vi "PlotOHparams.vi"() -> ()   [LabVIEW 2014]
uses:
  Slicer_11-28/LVslicer/Slice/TypeDefs/RectHatch.ctl
  Slicer_11-28/LVslicer/Slice/TypeDefs/PowerSpeed.ctl
  Slicer_11-28/LVslicer/Slice/TypeDefs/Area PWRMap Params.ctl
  <vilib>/picture/3D Picture Control/Object/Create Object (name).vi
  <vilib>/Utility/file.llb/Read From Spreadsheet File (DBL).vi
  <vilib>/picture/3D Picture Control/NI_3D Picture Control.lvlib
panel:
  out "Array":T1[](array[typedef])
  out "Layer":dbl
  in  "stop":bool
  out "3D Picture":refnum<vi>(3d-picture)
  out "OH":T2(array[cluster])=[{-30.0, 30.0, 382.0, 300.0, 114.6, 229.2, 229.2, 382.0, 382.0}, {-15.0, 30.0, 382.0, 300.0, 95.5, 191.0, 286.5, 382.0, 382.0}, {0.0, 30.0, 327.0, 150.0, 98.1, 196.2, 196.2, 327.0, 327.0}, {15.0, 30.0, 382.0, 300.0, 114.6, 229.2, 229.2, 382.0, 382.0}, {30.0, 30.0, 382.0, 300.0, 152.8, 191.0, 229.2, 267.4, 382.0}, {-30.0, 15.0, 382.0, 300.0, 95.5, 191.0, 286.5, 382.0, 382.0}, {-15.0, 15.0, 327.0, 150.0, 81.75, 163.5, 245.25, 327.0, 327.0}, {0.0, 15.0, 382.0, 300.0, 152.8, 191.0, 229.2, 267.4, 382.0}, {15.0, 15.0, 327.0, 150.0, 130.8, 163.5, 196.2, 228.9, 327.0}, {30.0, 15.0, 382.0, 300.0, 114.6, 229.2, 229.2, 382.0, 382.0}, {-30.0, 0.0, 327.0, 150.0, 98.1, 196.2, 196.2, 327.0, 327.0}, {-15.0, 0.0, 382.0, 300.0, 95.5, 191.0, 286.5, 382.0, 382.0}, {0.0, 0.0, 327.0, 150.0, 81.75, 163.5, 245.25, 327.0, 327.0}, {15.0, 0.0, 382.0, 300.0, 152.8, 191.0, 229.2, 267.4, 382.0}, {30.0, 0.0, 327.0, 150.0, 130.8, 163.5, 196.2, 228.9, 327.0}, {-30.0, -15.0, 382.0, 300.0, 114.6, 229.2, 229.2, 382.0, 382.0}, {-15.0, -15.0, 327.0, 150.0, 98.1, 196.2, 196.2, 327.0, 327.0}, {0.0, -15.0, 382.0, 300.0, 95.5, 191.0, 286.5, 382.0, 382.0}, {15.0, -15.0, 327.0, 150.0, 81.75, 163.5, 245.25, 327.0, 327.0}, {30.0, -15.0, 382.0, 300.0, 152.8, 191.0, 229.2, 267.4, 382.0}, {-30.0, -30.0, 382.0, 300.0, 114.6, 229.2, 229.2, 382.0, 382.0}, {-15.0, -30.0, 382.0, 300.0, 95.5, 191.0, 286.5, 382.0, 382.0}, {0.0, -30.0, 327.0, 150.0, 130.8, 163.5, 196.2, 228.9, 327.0}, {15.0, -30.0, 382.0, 300.0, 152.8, 191.0, 229.2, 267.4, 382.0}, {30.0, -30.0, 327.0, 150.0, 98.1, 196.2, 196.2, 327.0, 327.0}]
  in  "DummyCubeLoc":cluster{dbl, dbl}={-45.0, 30.0}
  in  "Save?":bool
  in  "Path":path=path "C:/Users/deane1/Documents/GitHub/TestRuns"
  in  "HighPower":dbl=500.0
  in  "Display":T3={"Mode"=enum."Inherit Value", "PointSize"=1.0, "LineWidth"=1.0}
  in  "LayerEnd":u32=170
  in  "LayerStart":u32=170
  in  "HatchPow":T4={"Power"=300.0, "Mark Speed"=400.0, "Jump Speed"=1000.0}
  in  "RectHatch":T5={"Width"=10.0, "Height"=10.0, "Angle"=45.0, "OffX"=0.1, "OffY"=0.1, "Spacing"=0.1} {"Spacing" format="%#_13g"; "OffY" format="%#_13g"; "OffX" format="%#_13g"; "Height" format="%#_13g"; "Width" format="%#_13g"}
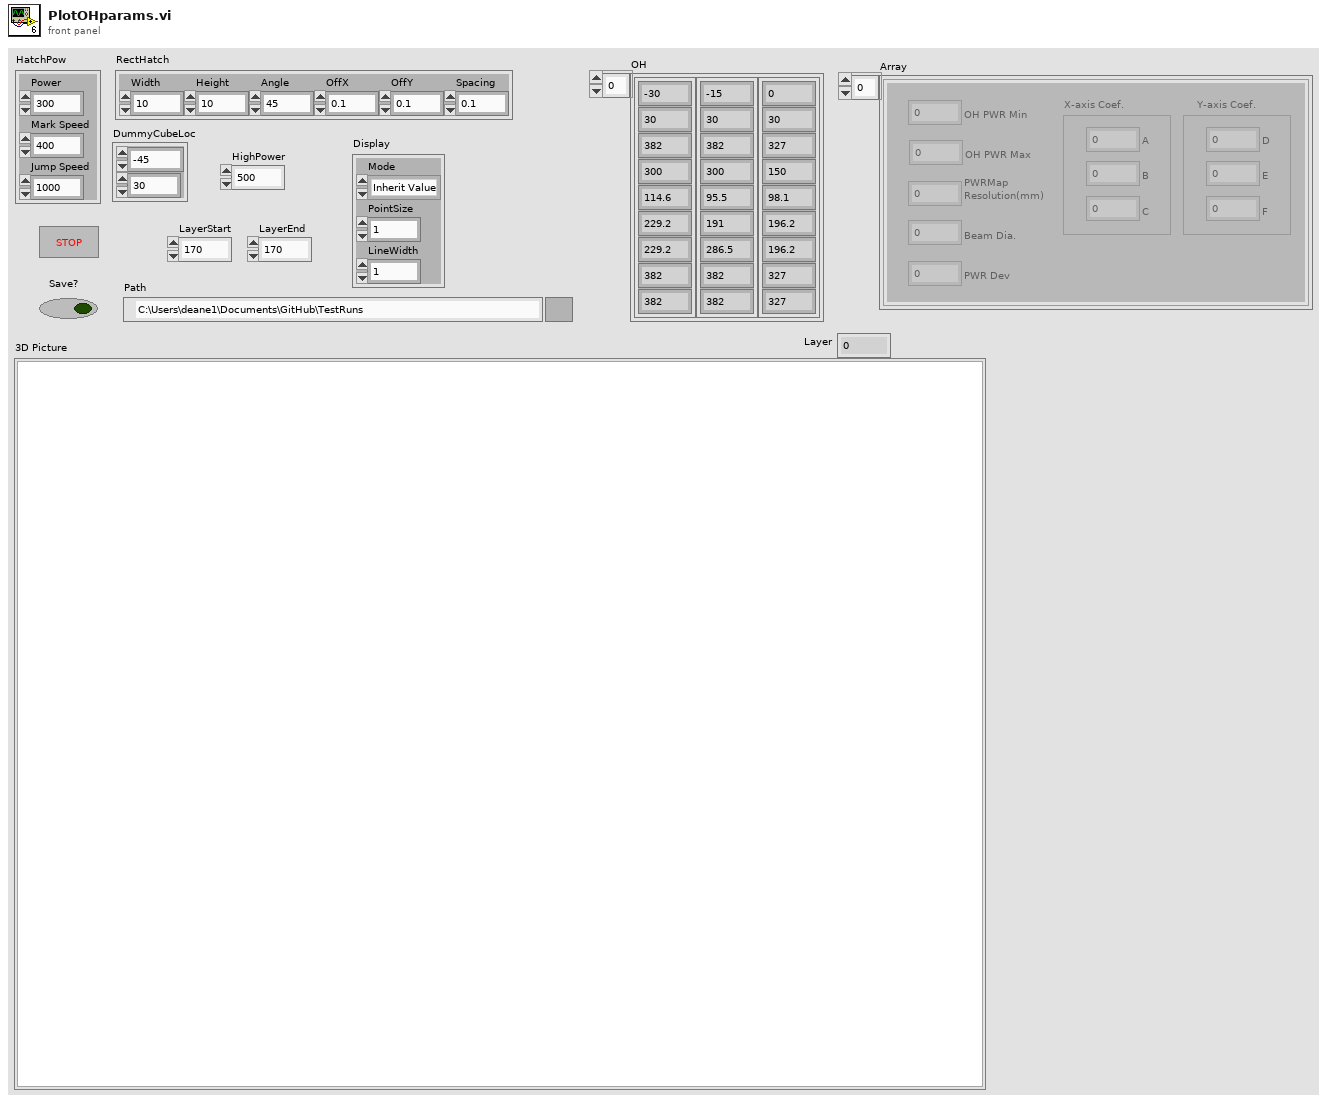
[diagram p1: front panel]
types:
  T1 = typedef "Area PWRMap Params.ctl" = cluster{"PWRMap \nResolution(mm)":dbl, "Beam Dia.":sgl, "PWR Dev":u32, "OH PWR Min":dbl, "X-axis Coef.":cluster{"A":dbl, "B":dbl, "C":dbl}, "OH PWR Max":dbl, "Y-axis Coef.":cluster{"D":dbl, "E":dbl, "F":dbl}}
  T2 = cluster{dbl, dbl, dbl, dbl, dbl, dbl, dbl, dbl, dbl}[]
  T3 = cluster{"Mode":enum16{"Inherit Value", "Points", "Wireframe", "Polygons"}, "PointSize":sgl, "LineWidth":sgl}
  T4 = typedef "PowerSpeed.ctl" = cluster{"Power":dbl, "Mark Speed":dbl, "Jump Speed":dbl}
  T5 = typedef "RectHatch.ctl" = cluster{"Width":dbl, "Height":dbl, "Angle":sgl, "OffX":dbl, "OffY":dbl, "Spacing":dbl}
  T6 = cluster{dbl, dbl, dbl, dbl, dbl, dbl, dbl, dbl, dbl}
  T7 = typedef "PathSupreme.ctl" = cluster{"VelocityProfiles":T8[], "Path":T9}
  T8 = typedef "VelocityProfile.ctl" = cluster{"ID":u32, "Velocity":dbl, "Mode":string, "tV1":u32, "tV2":u32, "tL1":u32, "tL2":u32}
  T9 = typedef "PathCut.ctl" = cluster{"Type":string, "Tag":string, "Segments":T10[]}
  T10 = typedef "Segment.ctl" = cluster{"SegmentID":u16, "Power":sgl, "idxVelocityProfile":u16, "End":cluster{"X":sgl, "Y":sgl}}
  T11 = typedef "Point3D.ctl" = cluster{"X":sgl, "Y":sgl, "Z":sgl}
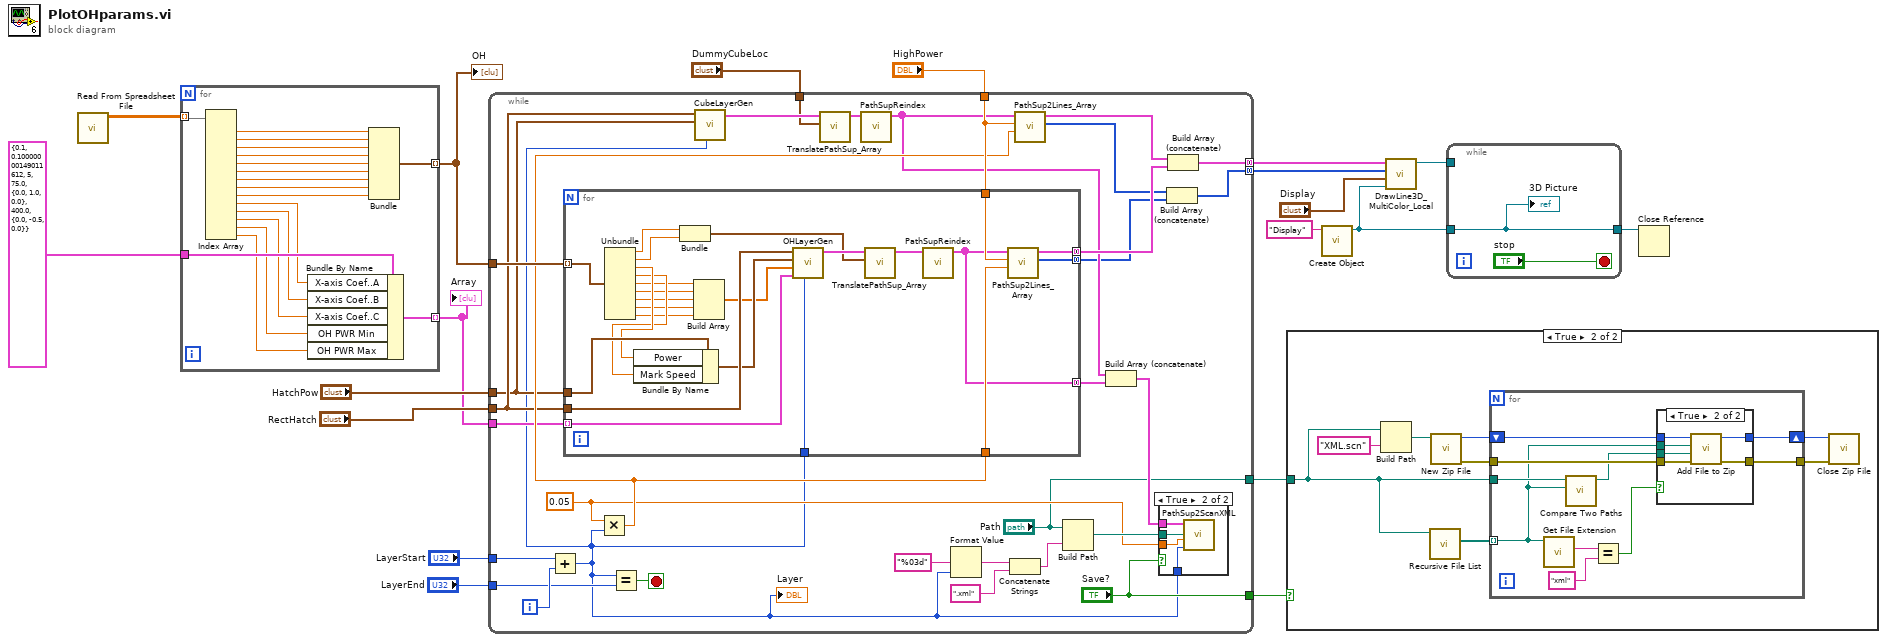
[diagram p0: block diagram]
diagram:
  n1 = call-poly <vilib>:"Read From Spreadsheet File.vi"() -> ("all rows"=w19:dbl[][])  [unwired: 7 in, 4 out]
  n2 = for {
    tunnel: w19 -> [w37] mode=indexing
    tunnel: [w32] -> w17 mode=indexing
    tunnel: T1 {"PWRMap \nResolution(mm)"=0.1, "Beam Dia."=0.1, "PWR Dev"=5, "OH PWR Min"=75.0, "X-axis Coef."={"A"=0.0, "B"=1.0, "C"=0.0}, "OH PWR Max"=400.0, "Y-axis Coef."={"D"=0.0, "E"=-0.5, "F"=0.0}} ("OH Power Map  Params (mm, Watts)") -> [w26]
    tunnel: [w22] -> w11 mode=indexing
    n3 = Index Array(array=w37) -> (element #1=w35:dbl, element #2=w36:dbl, element #3=w34:dbl, element #4=w33:dbl, element #5=w31:dbl, element #6=w30:dbl, element #7=w29:dbl, element #8=w28:dbl, element #9=w27:dbl, element #10=w23:dbl, element #11=w24:dbl, element #12=w25:dbl, element #13=w21:dbl, element #14=w20:dbl)  [unwired: 14 in]
    n4 = Bundle By Name(cluster=w26, "X-axis Coef..A"=w23, "X-axis Coef..B"=w24, "X-axis Coef..C"=w25, "OH PWR Min"=w21, "OH PWR Max"=w20) -> (w22:T1)
    n5 = Bundle(w35, w36, w34, w33, w31, w30, w29, w28, w27) -> (w32:T6)  [unwired: 1 in]
  }
  "OH" <- w17
  "Array" <- w11
  n6 = while {
    tunnel: "HighPower" -> [w56]
    tunnel: [w48] -> w10 mode=concatenating
    tunnel: [w53] -> w9 mode=concatenating
    tunnel: w17 -> [w66]
    tunnel: "RectHatch" -> [w51]
    tunnel: "HatchPow" -> [w50]
    tunnel: "LayerEnd" -> [w65]
    tunnel: "LayerStart" -> [w64]
    tunnel: "DummyCubeLoc" -> [w57]
    tunnel: w11 -> [w49]
    tunnel: ["Path"] -> w4
    tunnel: ["Save?"] -> w2
    i -> [w68]
    stop <- w67 stop-if-true
    w43 = 0.05 ("y")
    n7 = Add(x=w64, y=w68) -> (x+y=w40:u32)
    "Layer" <- w40
    n8 = Multiply(x=w43, y=w40) -> (x*y=w55:dbl)
    n9 = for {
      tunnel: w40 -> [w96]
      tunnel: w55 -> [w90]
      tunnel: w56 -> [w87]
      tunnel: [w95] -> w54 mode=concatenating
      tunnel: w66 -> [w94] mode=indexing
      tunnel: w51 -> [w93]
      tunnel: w50 -> [w85]
      tunnel: [w73] -> w52 mode=concatenating
      tunnel: [w86] -> w39 mode=concatenating
      tunnel: w49 -> [w75] mode=indexing
      n10 = Unbundle(w94) -> (w92:dbl, w91:dbl, w83:dbl, w82:dbl, w81:dbl, w80:dbl, w79:dbl, w78:dbl, w77:dbl)
      n11 = Bundle By Name(cluster=w85, "Power"=w83, "Mark Speed"=w82) -> (w84:T4)
      n12 = Bundle(w92, w91) -> (w88:cluster{dbl, dbl})  [unwired: 1 in]
      n13 = Build Array(w81, w80, w79, w78, w77) -> (w76:dbl[])
      n14 = call "OHLayerGen.vi"("Layer"=w96, "OH Power Map \nParams (mm, Watts)"=w75, "OHpows"=w76, "HatchPow"=w84, "RectHatch"=w93) -> ("PathSups"=w89:T7[])  [unwired: 6 in]
      n15 = call "TranslatePathSup_Array.vi"("Offset"=w88, "PathSupsIn"=w89) -> ("PathSupsOut"=w74:T7[])  [unwired: 9 in]
      n16 = call "PathSupReindex.vi"("PathSupremes"=w74) -> ("PathSupOut"=w73:T7[])  [unwired: 10 in]
      n17 = call "PathSup2Lines_Array.vi"("Z"=w90, "HighPower"=w87, "PathSupIn"=w73) -> ("Colors"=w86:u32[], "Lines"=w95:cluster{"P0":T11, "P1":T11}[])  [unwired: 7 in]
    }
    n18 = Equal?(x=w40, y=w65) -> (x = y?=w67:bool)
    n19 = call "CubeLayerGen.vi"("Layer"=w40, "HatchPow"=w50, "RectHatch"=w51) -> ("PathSups"=w58:T7[])  [unwired: 8 in]
    n20 = call "TranslatePathSup_Array.vi"("Offset"=w57, "PathSupsIn"=w58) -> ("PathSupsOut"=w45:T7[])  [unwired: 9 in]
    n21 = call "PathSupReindex.vi"("PathSupremes"=w45) -> ("PathSupOut"=w44:T7[])  [unwired: 10 in]
    n22 = Format Value(format string="%03d", value (0)=w40) -> (output string=w62:string)  [unwired: 1 in]
    n23 = Concatenate Strings(w62, ".xml" ("string")) -> (w60:string)
    n24 = call "PathSup2Lines_Array.vi"("Z"=w55, "HighPower"=w56, "PathSupIn"=w44) -> ("Colors"=w38:u32[], "Lines"=w47:cluster{"P0":T11, "P1":T11}[])  [unwired: 7 in]
    n25 = Build Path(base path="Path", name or relative path=w60) -> (appended path=w59:path)
    n26 = Build Array (concatenate)(w44, w52) -> (w46:T7[])
    n27 = case shown="True" "Save?" {
      tunnel: w46 -> [_ w72]
      tunnel: w59 -> [_ w71]
      tunnel: w43 -> [_ w70]
      tunnel: w40 -> [_ w69]
      frame False {
      }
      frame True {
        n28 = call "PathSup2ScanXML.vi"("PathSupremes"=w72, "Path"=w71, "Thickness"=w70, "layer"=w69) -> ()  [unwired: 4 in, 1 out]
      }
    }
    n29 = Build Array (concatenate)(w38, w39) -> (w53:u32[])
    n30 = Build Array (concatenate)(w47, w54) -> (w48:cluster{"P0":T11, "P1":T11}[])
  }
  n31 = case shown="True" w2 {
    tunnel: w4 -> [_ w104]
    frame False {
    }
    frame True {
      n32 = Build Path(base path=w104, name or relative path="XML.scn") -> (appended path=w97:path)
      n33 = call <vilib>:"Recursive File List.vi"("Folder Path"=w104) -> ("All Files in Dir"=w99:path[])  [unwired: 6 in, 4 out]
      n34 = call <vilib>:"New Zip File.vi"("target"=w97) -> ("error out"=w103:errorcluster, "zip file out"=w102:i64)  [unwired: 4 in, 1 out]
      n35 = for {
        shift-right: [w111] -> w100
        shift-left: w102 -> [w113]
        tunnel: w103 -> [w114]
        tunnel: [w112] -> w101
        tunnel: w99 -> [w106] mode=indexing
        tunnel: w104 -> [w107]
        n36 = call <vilib>:"Get File Extension.vi"("file"=w106) -> ("lowercase file extension"=w110:string)  [unwired: 7 in, 3 out]
        n37 = call <vilib>:"Compare Two Paths.vi"("Path 2"=w106, "Path 1"=w107) -> ("Relative Path from 1 to 2"=w105:path)  [unwired: 6 in, 3 out]
        n38 = Equal?(x=w110, y="xml") -> (x = y?=w108:bool)
        n39 = case shown="True" w108 {
          tunnel: w114 -> [w115 w122]
          tunnel: w113 -> [w116 w121]
          tunnel: [w115 w120] -> w112
          tunnel: [w116 w119] -> w111
          tunnel: w106 -> [_ w118]
          tunnel: w105 -> [_ w117]
          frame False {
          }
          frame True {
            n40 = call <vilib>:"Add File to Zip.vi"("error in (no error)"=w122, "destination path in zip"=w117, "source file path"=w118, "zip file in"=w121) -> ("error out"=w120:errorcluster, "zip file out"=w119:i64)  [unwired: 6 in]
          }
        }
      }
      n41 = call <vilib>:"Close Zip File.vi"("error in (no error)"=w101, "zip file in"=w100) -> ()  [unwired: 5 in, 1 out]
    }
  }
  n42 = call-poly <vilib>:"Create Object.vi"("Name"="Display") -> ("Scene:New Object"=w5:refnum<vi>)  [unwired: 9 in, 1 out]
  n43 = call "DrawLine3D_MultiColor_Local.vi"("Scene Object In"=w5, "Display"="Display", "Colors"=w9, "Lines"=w10) -> ("Scene Object Out"=w1:refnum<vi>)  [unwired: 7 in]
  n44 = while {
    tunnel: w5 -> [w124]
    tunnel: [w124] -> w6
    tunnel: w1 -> [_]
    stop <- "stop" stop-if-true
    "3D Picture" <- w124
  }
  n45 = Close Reference(reference=w6) -> ()  [unwired: 1 in, 1 out]
